vi "Equilibrium_Detector_subVI.vi"(0 "Measurement Cluster In":T4, 1 "Raman Equil Threshold (counts)":dbl, 2 "Flow Equil Threshold (%)":dbl=100.0, 9 "Display Spectra?":bool) -> (4 "Equilibrium?":bool, 6 "Measurement Cluster Out":T4, 8 "Raman Equilibrium Display":T2(graph), 10 "Flow Equilibrium Display":T3(graph), 15 "Unfiltered and Filtered Flows Display":T1(graph))   [LabVIEW 2015]
uses:
  --Controls and TypeDefs--/Measurement_Cluster.ctl
  --Controls and TypeDefs--/Raman_Model_Data_Cluster.ctl
  <vilib>/ptbypt/NI_PtbyPt.lvlib
panel:
  # "Flow Rate Measurements"
  # "Temp Measurements"
  # "Raman Measurements"
  # "Flow Rate Measurements"
  # "Temp Measurements"
  # "Raman Measurements"
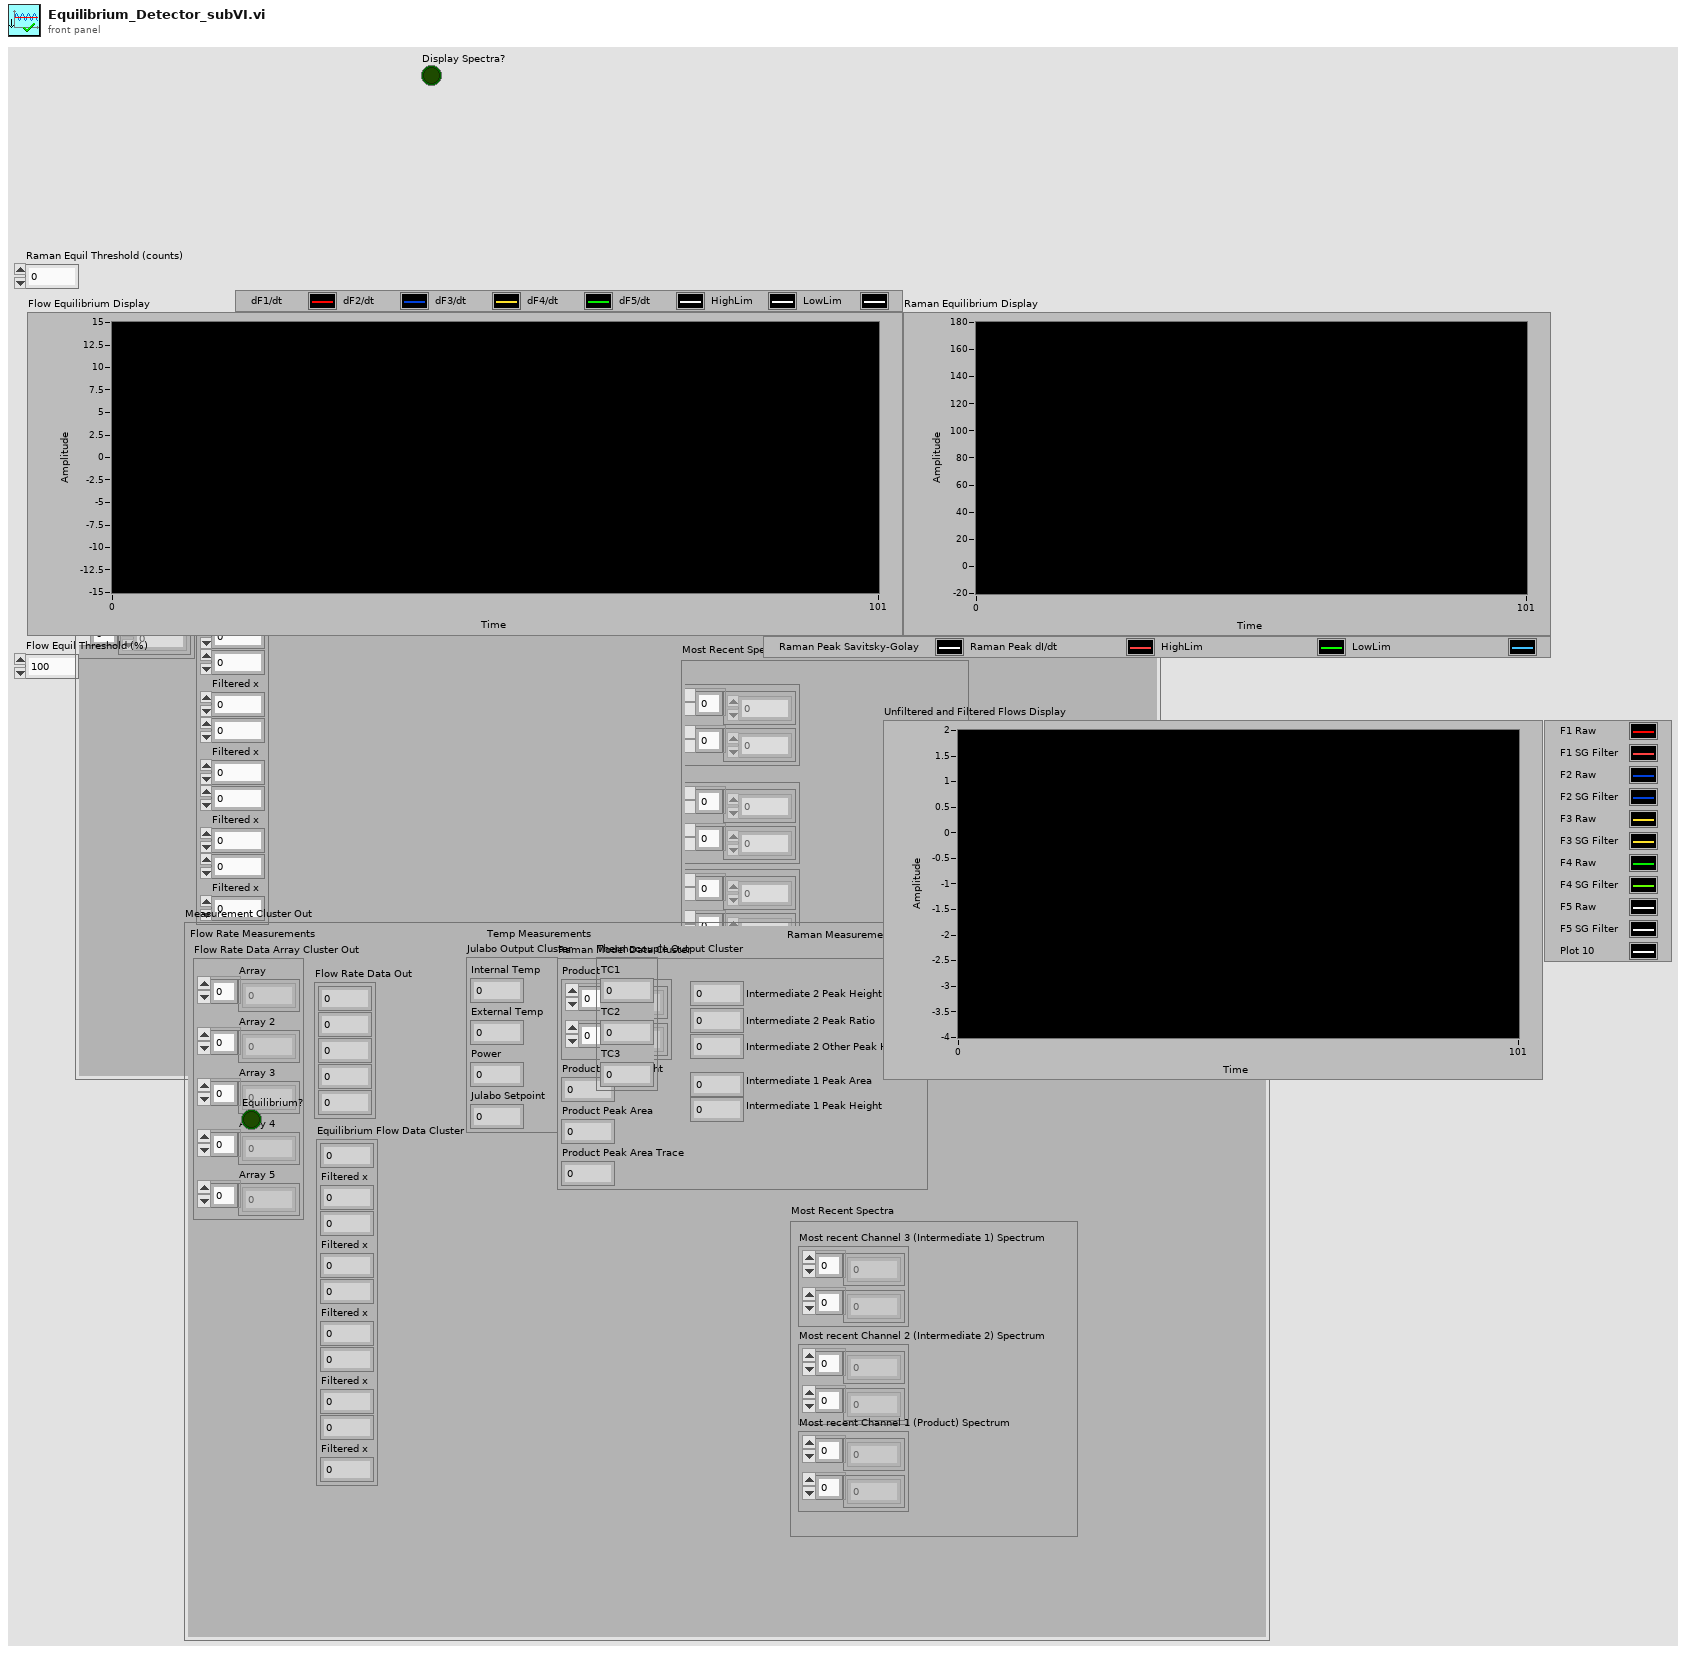
[diagram p1: front panel]
types:
  T1 = cluster{dbl, "Filtered x":dbl, dbl, "Filtered x":dbl, dbl, "Filtered x":dbl, dbl, "Filtered x":dbl, dbl, "Filtered x":dbl}
  T2 = cluster{"Filtered x":dbl, "dx/dt":dbl, "Raman Equil Threshold":dbl, dbl}
  T3 = cluster{"dx/dt":dbl, "dx/dt":dbl, "dx/dt":dbl, "dx/dt":dbl, "dx/dt":dbl, "Flow Equil Threshold":dbl, dbl}
  T4 = typedef "Measurement_Cluster.ctl" = cluster{"Raman Model Data Cluster":T5, "Julabo Output Cluster":cluster{"Internal Temp":dbl, "External Temp":dbl, "Power":i8, "Julabo Setpoint":dbl}, "Thermocouple Output Cluster":cluster{"TC1":dbl, "TC2":dbl, "TC3":dbl}, "Flow Rate Data Array Cluster Out":cluster{"Array":dbl[], "Array 2":dbl[], "Array 3":dbl[], "Array 4":dbl[], "Array 5":dbl[]}, "Flow Rate Data Out":cluster{dbl, dbl, dbl, dbl, dbl}, "Equilibrium?":bool, "Equilibrium Flow Data Cluster":cluster{dbl, "Filtered x":dbl, dbl, "Filtered x":dbl, dbl, "Filtered x":dbl, dbl, "Filtered x":dbl, dbl, "Filtered x":dbl}, "Most Recent Spectra":cluster{"Most recent Channel 3 (Intermediate 1) Spectrum":cluster{i32[], i32[]}, "Most recent Channel 2 (Intermediate 2) Spectrum":cluster{i32[], i32[]}, "Most recent Channel 1 (Product) Spectrum":cluster{i32[], i32[]}}}
  T5 = typedef "Raman_Model_Data_Cluster.ctl" = cluster{"Product Spectrum":cluster{i32[], i32[]}, "Product Peak Height":i32, "Product Peak Area":i32, "Product Peak Area Trace":i32, "Intermediate 2 Peak Height":i32, "Intermediate 1 Peak Area":i32, "Intermediate 1 Peak Height":i32, "Intermediate 2 Other Peak Height":i32, "Intermediate 2 Peak Ratio":i32}
  T6 = cluster{"Array":dbl[], "Array 2":dbl[], "Array 3":dbl[], "Array 4":dbl[], "Array 5":dbl[]}
  T7 = cluster{dbl, dbl, dbl, dbl, dbl, "Flow Equil Threshold (%)":dbl, dbl}
  T8 = cluster{"Internal Temp":dbl, "External Temp":dbl, "Power":i8, "Julabo Setpoint":dbl}
  T9 = cluster{"Filtered x":dbl, "dx/dt":dbl, "Raman Equil Threshold (counts)":dbl, dbl}
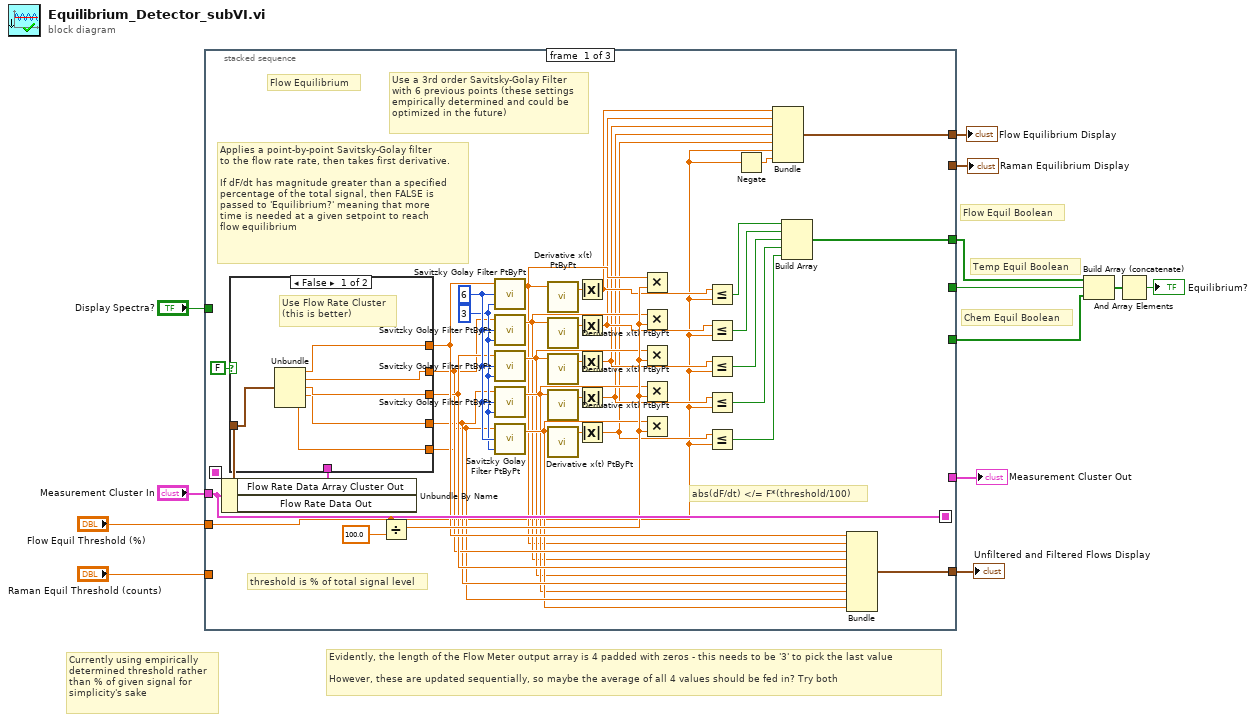
[diagram p0: block diagram]
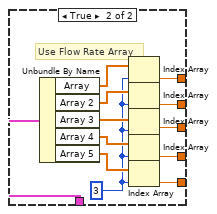
[diagram p2: hidden frame]
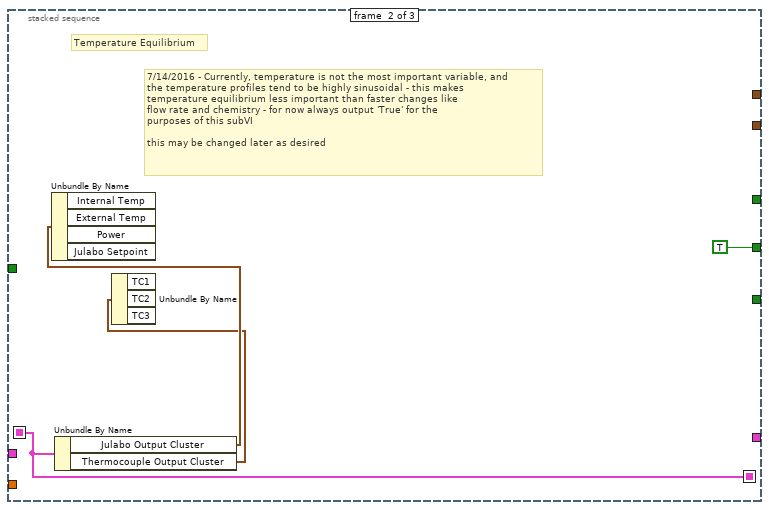
[diagram p3: hidden frame]
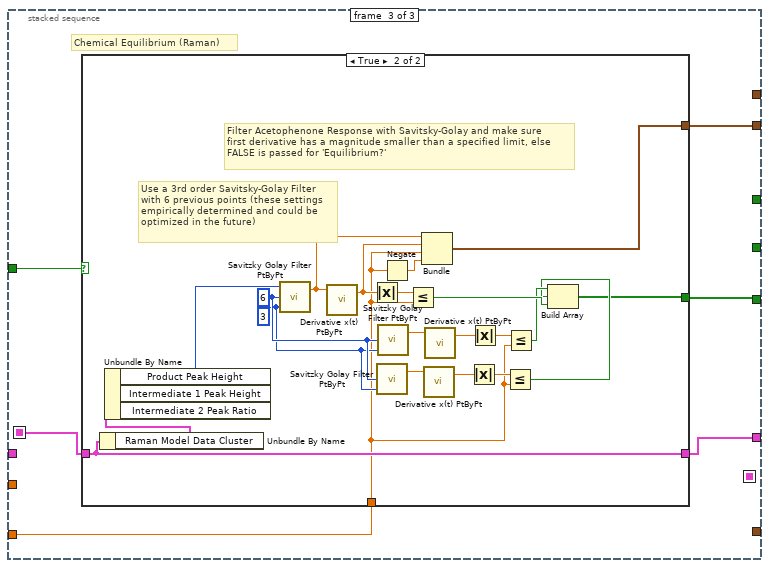
[diagram p4: hidden frame]
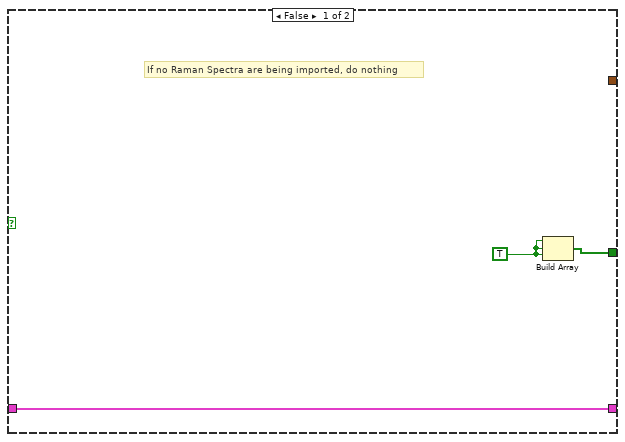
[diagram p5: hidden frame]
diagram:
  # "Currently using empirically\ndetermined threshold rather\nthan % of given signal for\nsimplicity's sake"
  # "Evidently, the length of the Flow Meter output array is 4 padded with zeros - this needs to be '3' to pick the last value\n\nHowever, these are updated sequentially, so maybe the average of all 4 values should be fed in? Try both"
  # "Chem Equil Boolean"
  # "Temp Equil Boolean"
  # "Flow Equil Boolean"
  n1 = stacked-sequence {
    seq-local: [w51 _ _] -> [_ w71 _]
    seq-local: [_ w71 _] -> [_ _ w78]
    tunnel: "Display Spectra?" -> [_ _ w79]
    tunnel: "Measurement Cluster In" -> [w51 _ _]
    tunnel: [_ _ w77] -> w11
    tunnel: [w50 _ _] -> w9
    tunnel: [_ TRUE _] -> w10
    tunnel: [w41 _ _] -> w6
    tunnel: "Flow Equil Threshold (%)" -> [w14 _ _]
    tunnel: "Raman Equil Threshold (counts)" -> [_ _ w76]
    tunnel: [_ _ w75] -> w3
    tunnel: [w22 _ _] -> w2
    tunnel: [_ _ w74] -> w1
    frame #0 {
      w48 = 3 ("order polynomial")
      w49 = 6 ("side points")
      # "Use a 3rd order Savitsky-Golay Filter\nwith 6 previous points (these settings\nempirically determined and could be\noptimized in the future)"
      # "abs(dF/dt) </= F*(threshold/100)"
      # "Applies a point-by-point Savitsky-Golay filter\nto the flow rate rate, then takes first derivative.\n\nIf dF/dt has magnitude greater than a specified\npercentage of the total signal, then FALSE is\npassed to 'Equilibrium?' meaning that more\ntime is needed at a given setpoint to reach\nflow equilibrium"
      # "threshold is % of total signal level"
      # "Flow Equilibrium"
      n2 = Unbundle By Name(w51) -> ("Flow Rate Data Array Cluster Out"=w47:T6, "Flow Rate Data Out"=w21:cluster{dbl, dbl, dbl, dbl, dbl})
      n3 = case shown="False" FALSE {
        tunnel: w47 -> [_ w65]
        tunnel: [w56 w62] -> w32
        tunnel: [w54 w61] -> w31
        tunnel: [w55 w60] -> w30
        tunnel: [w53 w59] -> w29
        tunnel: [w52 w58] -> w28
        tunnel: w21 -> [w57 _]
        frame False {
          # "Use Flow Rate Cluster\n(this is better)"
          n4 = Unbundle(w57) -> (w56:dbl, w55:dbl, w54:dbl, w53:dbl, w52:dbl)
        }
        frame True {
          w64 = 3 ("index")
          # "Use Flow Rate Array"
          n5 = Unbundle By Name(w65) -> ("Array"=w63:dbl[], "Array 2"=w66:dbl[], "Array 3"=w67:dbl[], "Array 4"=w68:dbl[], "Array 5"=w69:dbl[])
          n6 = Index Array(array=w63, index=w64) -> (element=w62:dbl)
          n7 = Index Array(array=w66, index=w64) -> (element=w60:dbl)
          n8 = Index Array(array=w67, index=w64) -> (element=w61:dbl)
          n9 = Index Array(array=w68, index=w64) -> (element=w59:dbl)
          n10 = Index Array(array=w69, index=w64) -> (element=w58:dbl)
        }
      }
      n11 = Divide(x=w14, y=100.0) -> (x/y=w34:dbl)
      n12 = call <vilib>:"Savitzky Golay Filter PtByPt.vi"("order polynomial"=w48, "side points"=w49, "x"=w32) -> ("Filtered x"=w23:dbl)  [unwired: 1 in, 1 out]
      n13 = call <vilib>:"Savitzky Golay Filter PtByPt.vi"("order polynomial"=w48, "side points"=w49, "x"=w30) -> ("Filtered x"=w24:dbl)  [unwired: 1 in, 1 out]
      n14 = call <vilib>:"Savitzky Golay Filter PtByPt.vi"("order polynomial"=w48, "side points"=w49, "x"=w31) -> ("Filtered x"=w25:dbl)  [unwired: 1 in, 1 out]
      n15 = call <vilib>:"Savitzky Golay Filter PtByPt.vi"("order polynomial"=w48, "side points"=w49, "x"=w29) -> ("Filtered x"=w26:dbl)  [unwired: 1 in, 1 out]
      n16 = call <vilib>:"Savitzky Golay Filter PtByPt.vi"("order polynomial"=w48, "side points"=w49, "x"=w28) -> ("Filtered x"=w27:dbl)  [unwired: 1 in, 1 out]
      n17 = call <vilib>:"Derivative x(t) PtByPt.vi"("x"=w23) -> ("dx/dt"=w36:dbl)  [unwired: 3 in, 1 out]
      n18 = call <vilib>:"Derivative x(t) PtByPt.vi"("x"=w24) -> ("dx/dt"=w37:dbl)  [unwired: 3 in, 1 out]
      n19 = call <vilib>:"Derivative x(t) PtByPt.vi"("x"=w25) -> ("dx/dt"=w38:dbl)  [unwired: 3 in, 1 out]
      n20 = call <vilib>:"Derivative x(t) PtByPt.vi"("x"=w26) -> ("dx/dt"=w39:dbl)  [unwired: 3 in, 1 out]
      n21 = call <vilib>:"Derivative x(t) PtByPt.vi"("x"=w27) -> ("dx/dt"=w40:dbl)  [unwired: 3 in, 1 out]
      n22 = Absolute Value(x=w36) -> (abs(x)=w19:dbl)
      n23 = Absolute Value(x=w37) -> (abs(x)=w18:dbl)
      n24 = Absolute Value(x=w38) -> (abs(x)=w17:dbl)
      n25 = Absolute Value(x=w39) -> (abs(x)=w16:dbl)
      n26 = Absolute Value(x=w40) -> (abs(x)=w15:dbl)
      n27 = Multiply(x=w23, y=w34) -> ()  [unwired: 1 out]
      n28 = Multiply(x=w24, y=w34) -> ()  [unwired: 1 out]
      n29 = Multiply(x=w25, y=w34) -> ()  [unwired: 1 out]
      n30 = Multiply(x=w26, y=w34) -> ()  [unwired: 1 out]
      n31 = Multiply(x=w27, y=w34) -> ()  [unwired: 1 out]
      n32 = Less Or Equal?(x=w19, y=w14) -> (x <= y?=w46:bool)
      n33 = Less Or Equal?(x=w18, y=w14) -> (x <= y?=w45:bool)
      n34 = Less Or Equal?(x=w17, y=w14) -> (x <= y?=w44:bool)
      n35 = Less Or Equal?(x=w16, y=w14) -> (x <= y?=w43:bool)
      n36 = Less Or Equal?(x=w15, y=w14) -> (x <= y?=w42:bool)
      n37 = Negate(x=w14) -> (-x=w33:dbl)
      n38 = Bundle(w19, w18, w17, w16, w15, "Flow Equil Threshold (%)"=w14, w33) -> (w41:T7)  [unwired: 1 in]
      n39 = Build Array(w46, w45, w44, w43, w42) -> (w50:bool[])
      n40 = Bundle(w32, "Filtered x"=w23, w30, "Filtered x"=w24, w31, "Filtered x"=w25, w29, "Filtered x"=w26, w28, "Filtered x"=w27) -> (w22:T1)  [unwired: 1 in]
    }
    frame #1 {
      # "7/14/2016 - Currently, temperature is not the most important variable, and \nthe temperature profiles tend to be highly sinusoidal - this makes\ntemperature equilibrium less important than faster changes like \nflow rate and chemistry - for now always output 'True' for the\npurposes of this subVI\n\nthis may be changed later as desired"
      # "Temperature Equilibrium"
      n41 = Unbundle By Name(w71) -> ("Julabo Output Cluster"=w73:T8, "Thermocouple Output Cluster"=w72:cluster{"TC1":dbl, "TC2":dbl, "TC3":dbl})
      n42 = Unbundle By Name(w73) -> ()  [unwired: 4 out]
      n43 = Unbundle By Name(w72) -> ()  [unwired: 3 out]
    }
    frame #2 {
      # "Chemical Equilibrium (Raman)"
      n44 = case shown="True" w79 {
        tunnel: w78 -> [w82 w103]
        tunnel: [w82 w103] -> w77
        tunnel: w76 -> [_ w83]
        tunnel: [w80 w92] -> w74
        tunnel: [_ w96] -> w75
        frame False {
          w81 = TRUE
          # "If no Raman Spectra are being imported, do nothing"
          n45 = Build Array(w81, w81, w81) -> (w80:bool[])
        }
        frame True {
          w90 = 3 ("order polynomial")
          w91 = 6 ("side points")
          # "Use a 3rd order Savitsky-Golay Filter\nwith 6 previous points (these settings\nempirically determined and could be\noptimized in the future)"
          # "Filter Acetophenone Response with Savitsky-Golay and make sure\nfirst derivative has a magnitude smaller than a specified limit, else\nFALSE is passed for 'Equilibrium?'"
          n46 = Unbundle By Name(w103) -> ("Raman Model Data Cluster"=w102:T5)
          n47 = Unbundle By Name(w102) -> ("Product Peak Height"=w101:i32)  [unwired: 2 out]
          n48 = call <vilib>:"Savitzky Golay Filter PtByPt.vi"("order polynomial"=w90, "side points"=w91, "x"=w101) -> ("Filtered x"=w100:dbl)  [unwired: 1 in, 1 out]
          n49 = call <vilib>:"Derivative x(t) PtByPt.vi"("x"=w100) -> ("dx/dt"=w99:dbl)  [unwired: 3 in, 1 out]
          n50 = Absolute Value(x=w99) -> (abs(x)=w98:dbl)
          n51 = call <vilib>:"Savitzky Golay Filter PtByPt.vi"("order polynomial"=w90, "side points"=w91) -> ("Filtered x"=w88:dbl)  [unwired: 2 in, 1 out]
          n52 = call <vilib>:"Savitzky Golay Filter PtByPt.vi"("order polynomial"=w90, "side points"=w91) -> ("Filtered x"=w89:dbl)  [unwired: 2 in, 1 out]
          n53 = Negate(x=w83) -> (-x=w97:dbl)
          n54 = Less Or Equal?(x=w98, y=w83) -> (x <= y?=w95:bool)
          n55 = Bundle("Filtered x"=w100, "dx/dt"=w99, "Raman Equil Threshold (counts)"=w83, w97) -> (w96:T9)  [unwired: 1 in]
          n56 = call <vilib>:"Derivative x(t) PtByPt.vi"("x"=w88) -> ("dx/dt"=w86:dbl)  [unwired: 3 in, 1 out]
          n57 = call <vilib>:"Derivative x(t) PtByPt.vi"("x"=w89) -> ("dx/dt"=w87:dbl)  [unwired: 3 in, 1 out]
          n58 = Absolute Value(x=w86) -> (abs(x)=w84:dbl)
          n59 = Absolute Value(x=w87) -> (abs(x)=w85:dbl)
          n60 = Less Or Equal?(x=w84, y=w83) -> (x <= y?=w93:bool)
          n61 = Less Or Equal?(x=w85, y=w83) -> (x <= y?=w94:bool)
          n62 = Build Array(w94, w93, w95) -> (w92:bool[])
        }
      }
    }
  }
  "Measurement Cluster Out" <- w11
  "Flow Equilibrium Display" <- w6
  "Raman Equilibrium Display" <- w3
  "Unfiltered and Filtered Flows Display" <- w2
  n63 = Build Array (concatenate)(w9, w10, w1) -> (w8:bool[])
  n64 = And Array Elements(Boolean array=w8) -> (logical AND=→"Equilibrium?":bool)
